vi "TestExample.vi"() -> ()   [LabVIEW 2013]
uses:
  Joystick_UserEvent.ctl
panel:
  out "x+1":i32
  out "Step":i32
  out "Direction 2":i32
  out "appended array 2":i32[](array[numeric])
  out "appended array":dbl[](array[numeric])
  out "Speed":dbl
  out "Direction":i32
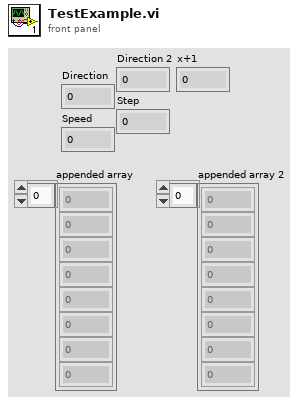
[diagram p1: front panel]
types:
  T1 = typedef "Joystick_UserEvent.ctl" = cluster{"StepMove":refnum<user-event>, "ContMove":refnum<user-event>, "EStop":refnum<user-event>}
  T2 = cluster{"axes total":u32, "buttons total":u32, "pov total":u32, "device name":string}[]
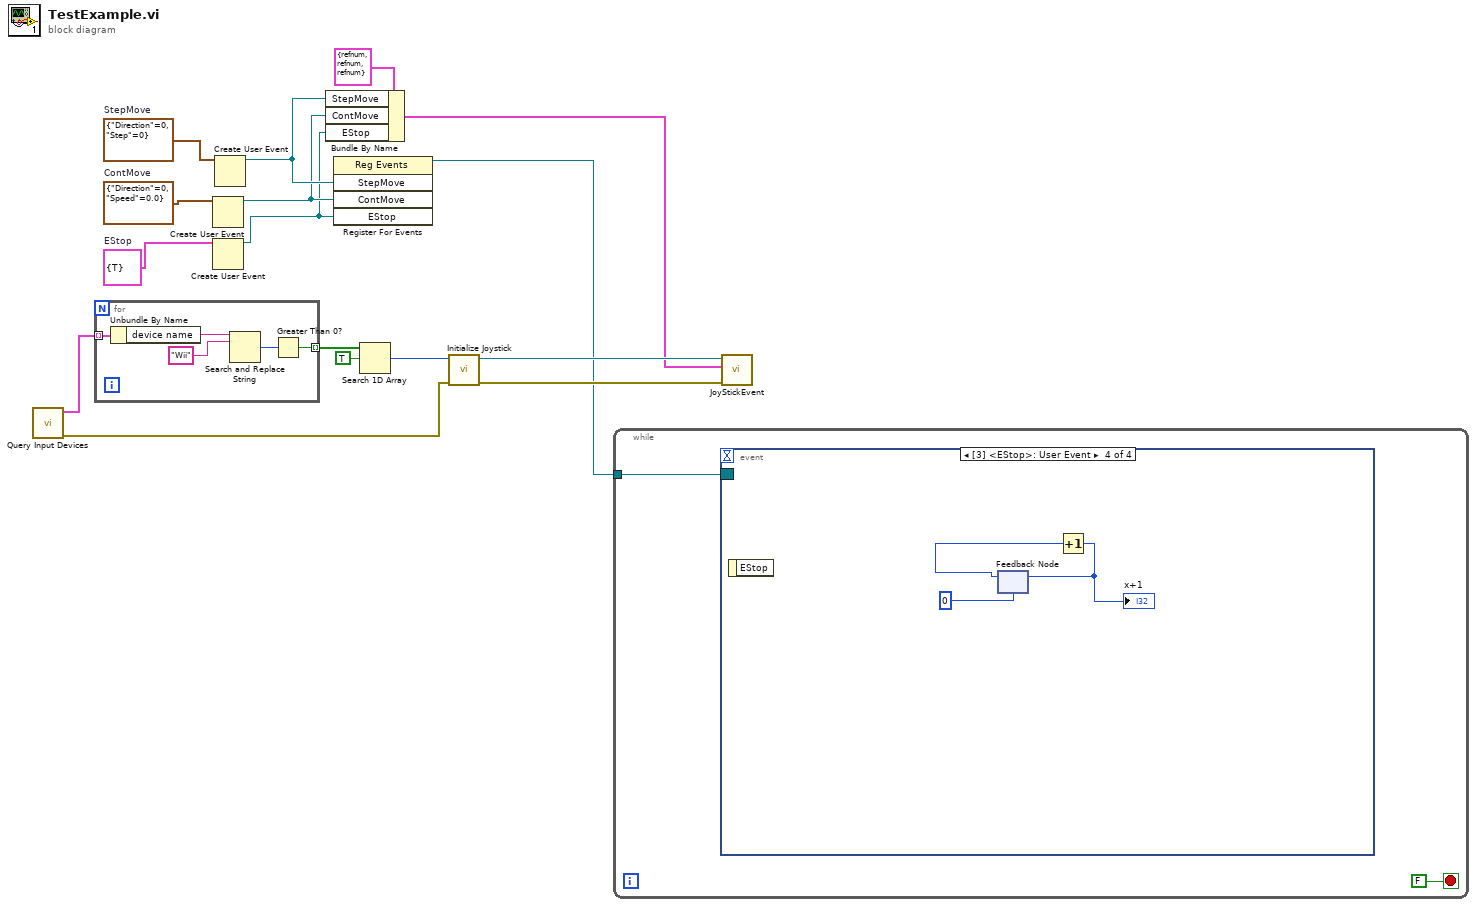
[diagram p0: block diagram]
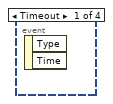
[diagram p2: hidden frame]
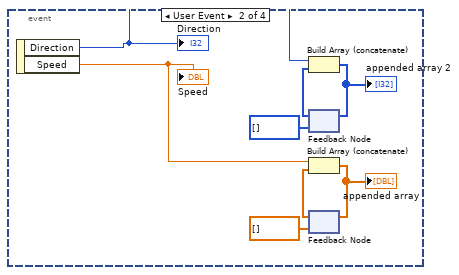
[diagram p3: hidden frame]
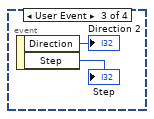
[diagram p4: hidden frame]
diagram:
  w7 = cluster{"EStop":bool} {"EStop"=TRUE}  # EStop
  w12 = cluster{"Direction":i32, "Speed":dbl} {"Direction"=0, "Speed"=0.0}  # ContMove
  w13 = cluster{"Direction":i32, "Step":i32} {"Direction"=0, "Step"=0}  # StepMove
  n1 = call <vilib>:"Query Input Devices.vi"() -> ("error out"=w16:errorcluster, "joystick info"=w4:T2)  [unwired: 8 in, 2 out]
  n2 = for {
    tunnel: w4 -> [w21] mode=indexing
    tunnel: [w17] -> w3 mode=indexing
    n3 = Unbundle By Name(w21) -> ("device name"=w20:string)
    n4 = Search and Replace String(input string=w20, search string="Wii") -> (number of replacements=w18:i32)  [unwired: 6 in, 3 out]
    n5 = Greater Than 0?(x=w18) -> (x > 0?=w17:bool)
  }
  n6 = Create User Event(user event datatype=w12) -> (user event=w10:refnum<user-event>)  [unwired: 1 in, 1 out]
  n7 = Create User Event(user event datatype=w7) -> (user event=w6:refnum<user-event>)  [unwired: 1 in, 1 out]
  n8 = Create User Event(user event datatype=w13) -> (user event=w11:refnum<user-event>)  [unwired: 1 in, 1 out]
  n9 = Bundle By Name(cluster=T1 {"StepMove"=refnum, "ContMove"=refnum, "EStop"=refnum}, "StepMove"=w11, "ContMove"=w10, "EStop"=w6) -> (w9:T1)
  n10 = register-events(w11, w10, w6) -> (reference out=w5:refnum<event-registration>)  [unwired: 2 in, 1 out]
  n11 = Search 1D Array(1D array=w3, element=TRUE) -> (index of element=w1:i32)  [unwired: 1 in]
  n12 = call <vilib>:"Initialize Joystick.vi"("error in (no error)"=w16, "device index"=w1) -> ("error out"=w15:errorcluster, "device ID"=w14:refnum<k1>)  [unwired: 8 in]
  n13 = while {
    tunnel: w5 -> [w23]
    stop <- FALSE stop-if-true
    n14 = event shown="[3] <EStop>: User Event" {
      selector: w23 -> [_ _ _ _]
      dyn-events: _ -> [_ _ _ _]
      timeout: _ -> [_ _ _ _]
      event Timeout {
        n15 = event-data() -> ()  [unwired: 1 in, 2 out]
      }
      event User Event {
        n16 = event-data() -> ("Direction"=w30:i32, "Speed"=w27:dbl)  [unwired: 1 in]
        "Direction" <- w30
        "Speed" <- w27
        n17 = feedback #1(i32[] []) -> (w31:i32[])
        n18 = Build Array (concatenate)(w30, w31) -> (w29:i32[])
        "appended array 2" <- w29
        n19 = feedback-in #1(w29) -> ()
        n20 = feedback #2(dbl[] []) -> (w26:dbl[])
        n21 = Build Array (concatenate)(w27, w26) -> (w28:dbl[])
        "appended array" <- w28
        n22 = feedback-in #2(w28) -> ()
      }
      event User Event {
        n23 = event-data() -> ("Direction"=→"Direction 2":i32, "Step"=→"Step":i32)  [unwired: 1 in]
      }
      event User Event {
        n24 = event-data() -> ()  [unwired: 1 in, 1 out]
        n25 = feedback #3(0) -> (w35:i32)
        n26 = Increment(x=w35) -> (x+1=w34:i32)
        "x+1" <- w34
        n27 = feedback-in #3(w34) -> ()
      }
    }
  }
  n28 = call "JoyStickEvent.vi"("error in"=w15, "UserEvent_Handle"=w9, "device ID"=w14) -> ()  [unwired: 9 in]
